vi "GEA2 Script_Parse Read and Write.vi"(0 "Data":string) -> (4 "Expected Response":string, 8 "GEA2 Message":T1 {"Command" format="%02x"; "Destination" format="%02x"; "Source" format="%02x"})   [LabVIEW 2023]
uses:
  LabVIEW GEA2 Toolkit/GEA3/type defs/Data In.ctl
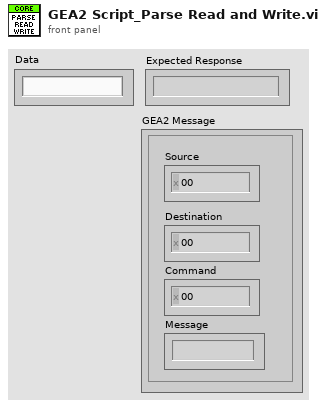
[diagram p1: front panel]
types:
  T1 = typedef "Data In.ctl" = cluster{"Source":u8, "Destination":u8, "Command":u8, "Message":string}
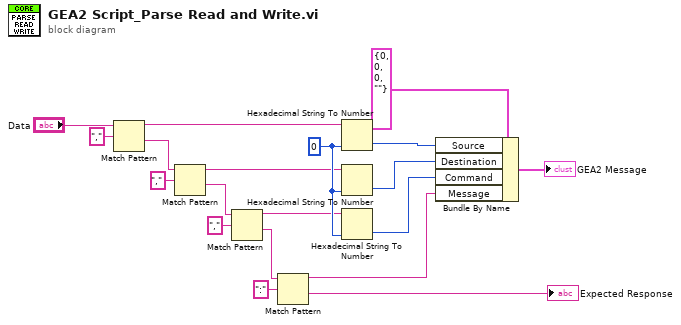
[diagram p0: block diagram]
diagram:
  w10 = u8 0
  n1 = Match Pattern(string="Data", regular expression=",") -> (before substring=w13:string, after substring=w12:string)  [unwired: 1 in, 2 out]
  n2 = Match Pattern(string=w12, regular expression=",") -> (before substring=w9:string, after substring=w7:string)  [unwired: 1 in, 2 out]
  n3 = Match Pattern(string=w7, regular expression=",") -> (before substring=w8:string, after substring=w6:string)  [unwired: 1 in, 2 out]
  n4 = Match Pattern(string=w6, regular expression=":") -> (before substring=w3:string, after substring=→"Expected Response":string)  [unwired: 1 in, 2 out]
  n5 = Hexadecimal String To Number(string=w13, default (0uL)=w10) -> (number=w11:u8)  [unwired: 1 in, 1 out]
  n6 = Hexadecimal String To Number(string=w9, default (0uL)=w10) -> (number=w4:u8)  [unwired: 1 in, 1 out]
  n7 = Hexadecimal String To Number(string=w8, default (0uL)=w10) -> (number=w5:u8)  [unwired: 1 in, 1 out]
  n8 = Bundle By Name(cluster=T1 {"Source"=0, "Destination"=0, "Command"=0, "Message"=""} ("Data In"), "Source"=w11, "Destination"=w4, "Command"=w5, "Message"=w3) -> (→"GEA2 Message":T1)
